vi "find_check_point.vi"(11 "input queue":string="DataFlow") -> ()   [LabVIEW 2016]
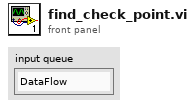
[diagram p1: front panel]
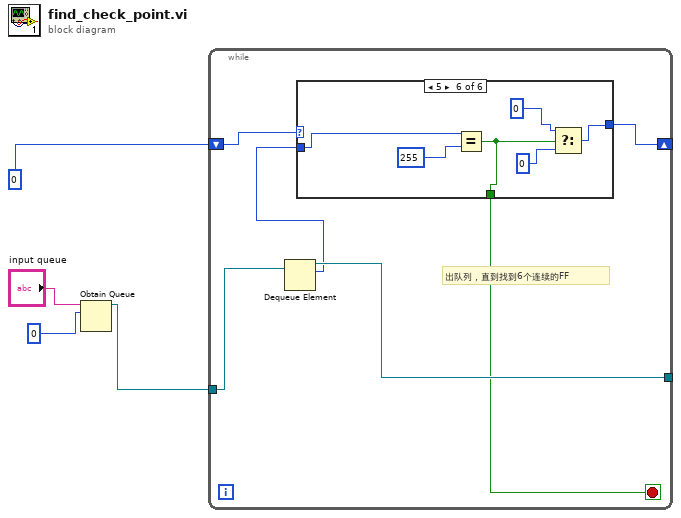
[diagram p0: block diagram]
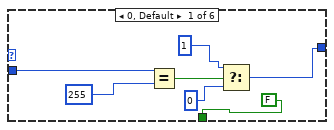
[diagram p2: hidden frame]
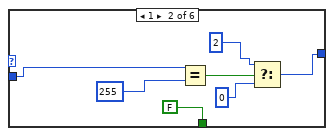
[diagram p3: hidden frame]
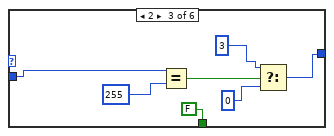
[diagram p4: hidden frame]
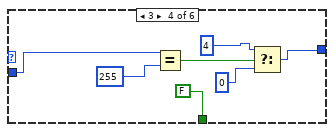
[diagram p5: hidden frame]
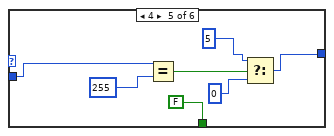
[diagram p6: hidden frame]
diagram:
  n1 = Obtain Queue(name (unnamed)="input queue", element data type=u8 0) -> (queue out=w1:refnum<queue>)  [unwired: 3 in, 2 out]
  n2 = while {
    tunnel: w1 -> [w10]
    tunnel: [w9] -> _
    shift-right: [w7] -> _
    shift-left: 0 -> [w8]
    stop <- w5 stop-if-true
    # "出队列，直到找到6个连续的FF"
    n3 = Dequeue Element(queue=w10) -> (queue out=w9:refnum<queue>, element=w6:u8)  [unwired: 2 in, 2 out]
    n4 = case shown="5" w8 {
      tunnel: [w12 w19 w27 w32 w39 w47] -> w7
      tunnel: w6 -> [w15 w20 w28 w34 w41 w48]
      tunnel: [FALSE FALSE FALSE FALSE FALSE w46] -> w5
      frame 0, Default {
        n5 = Equal?(x=w15, y=255) -> (x = y?=w16:bool)
        n6 = Select(t=1, s=w16, f=0) -> (s? t:f=w12:i32)
      }
      frame 1 {
        n7 = Equal?(x=w20, y=255) -> (x = y?=w23:bool)
        n8 = Select(t=2, s=w23, f=0) -> (s? t:f=w19:i32)
      }
      frame 2 {
        n9 = Equal?(x=w28, y=255) -> (x = y?=w26:bool)
        n10 = Select(t=3, s=w26, f=0) -> (s? t:f=w27:i32)
      }
      frame 3 {
        n11 = Equal?(x=w34, y=255) -> (x = y?=w38:bool)
        n12 = Select(t=4, s=w38, f=0) -> (s? t:f=w32:i32)
      }
      frame 4 {
        n13 = Equal?(x=w41, y=255) -> (x = y?=w42:bool)
        n14 = Select(t=5, s=w42, f=0) -> (s? t:f=w39:i32)
      }
      frame 5 {
        n15 = Equal?(x=w48, y=255) -> (x = y?=w46:bool)
        n16 = Select(t=0, s=w46, f=0) -> (s? t:f=w47:i32)
      }
    }
  }
